vi "Create MQTT Client.vi"(5 "Client in":refnum<class "Client.lvclass">, 8 "error in (no error)":errorcluster, 11 "ID (empty:generate new)":string) -> (0 "error out":errorcluster, 3 "Client out":refnum<class "Client.lvclass">)   [LabVIEW 2013, in "MQTT Server.lvlib" / "Client.lvclass"]
uses:
  Client.lvclass
  Control Packets/CONNACK/Connect Return Code -- enum.ctl
  Control Packets/PUBLISH/PUBLISH.lvclass
  Client.lvclass/Client.ctl
  Control Packets/ControlPacket/ControlPacket.lvclass
  Control Packets/CONNACK/CONNACK.lvclass
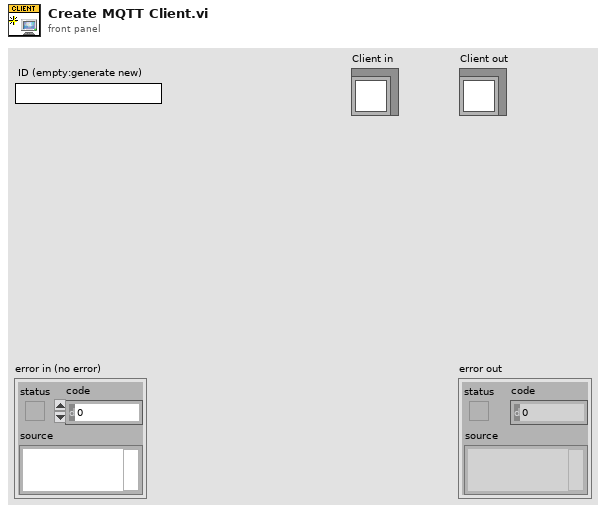
[diagram p1: front panel]
types:
  T1 = typedef "CONNACK.lvclass/Connect Return Code -- enum.ctl" = enum16{"Connection accepted", "Unacceptable protocol version", "Identifier Rejected", "Server Unavailable", "Bad Username or Password", "Not Authorized"}
  T2 = cluster{"Connection Status":refnum<user-event>, "Connected":refnum<user-event>, "Application Message":refnum<user-event>}
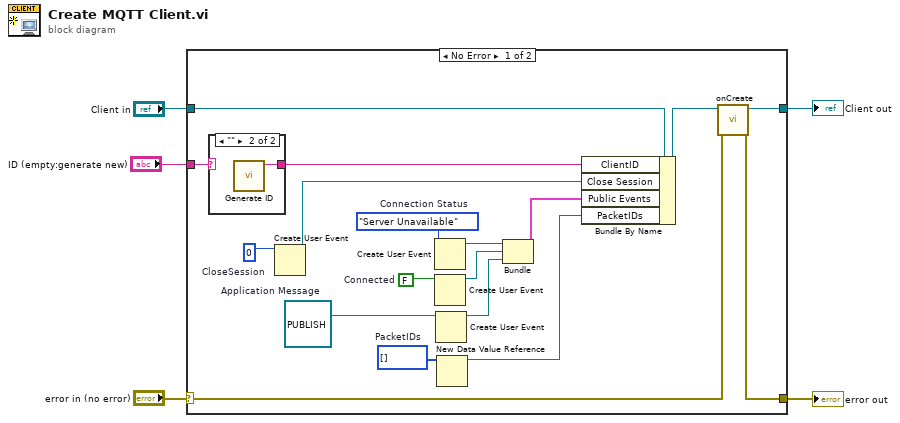
[diagram p0: block diagram]
diagram:
  n1 = case shown="No Error" "error in (no error)" {
    selector: "error in (no error)" -> [w18 w27]
    tunnel: [w17 w27] -> w1
    tunnel: [w19 w26] -> w2
    tunnel: "Client in" -> [w23 w26]
    tunnel: "ID (empty:generate new)" -> [w22 _]
    frame No Error {
      w7 = u16[] []  # PacketIDs
      w9 = refnum<class "PUBLISH.lvclass"> refnum  # Application Message
      w10 = FALSE  # Connected
      w12 = Connect_Return_Code_--_enum."Server Unavailable"  # Connection Status
      w16 = 0  # CloseSession
      n2 = case shown="\"\"" w22 {
        selector: w22 -> [w24 _]
        tunnel: [w24 w25] -> w21
        frame Default {
        }
        frame "" {
          n3 = call "Generate ID.vi"() -> ("ID"=w25:string)  [unwired: 11 in]
        }
      }
      n4 = Create User Event(user event datatype=w16) -> (user event=w15:refnum<user-event>)  [unwired: 1 in, 1 out]
      n5 = Create User Event(user event datatype=w12) -> (user event=w14:refnum<user-event>)  [unwired: 1 in, 1 out]
      n6 = Create User Event(user event datatype=w10) -> (user event=w11:refnum<user-event>)  [unwired: 1 in, 1 out]
      n7 = Create User Event(user event datatype=w9) -> (user event=w8:refnum<user-event>)  [unwired: 1 in, 1 out]
      n8 = New Data Value Reference(data value=w7) -> (data value reference=w6:refnum<data-value>)  [unwired: 1 in, 1 out]
      n9 = Bundle("Connection Status"=w14, "Connected"=w11, "Application Message"=w8) -> (w13:T2)  [unwired: 1 in]
      n10 = Bundle By Name(cluster=w23, "ClientID"=w21, "Close Session"=w15, "Public Events"=w13, "PacketIDs"=w6) -> (w20:refnum<class "Client.lvclass">)
      n11 = call-dynamic "onCreate.vi"("error in (no error)"=w18, "MQTT_Base in"=w20) -> ("error out"=w17:errorcluster, "MQTT_Base out"=w19:refnum<class "Client.lvclass">)  [unwired: 8 in]
    }
    frame Error {
    }
  }
  "error out" <- w1
  "Client out" <- w2
